vi "Load Slave Configuration.vi"(8 "error in":errorcluster) -> (0 "error out":errorcluster, 1 "JointMapping":T1, 2 "hw interface":T4, 3 "kinematic parameters":T3)   [LabVIEW 2013]
uses:
  <vilib>/robotics/Kinematics/Link/Joint Type.ctl
  Telemanipulation/Grips Robot/JointMapping.ctl
  <vilib>/NI/GXML/_subVIs/GXML SearchParser/Search Parser.vi
  <vilib>/NI/GXML/GXML.lvlib
  <vilib>/robotics/Kinematics/Link/NI_Robotics_Link.lvclass
  Telemanipulation/Grips Robot/Grips Robot.lvclass
panel:
  out "file path":path
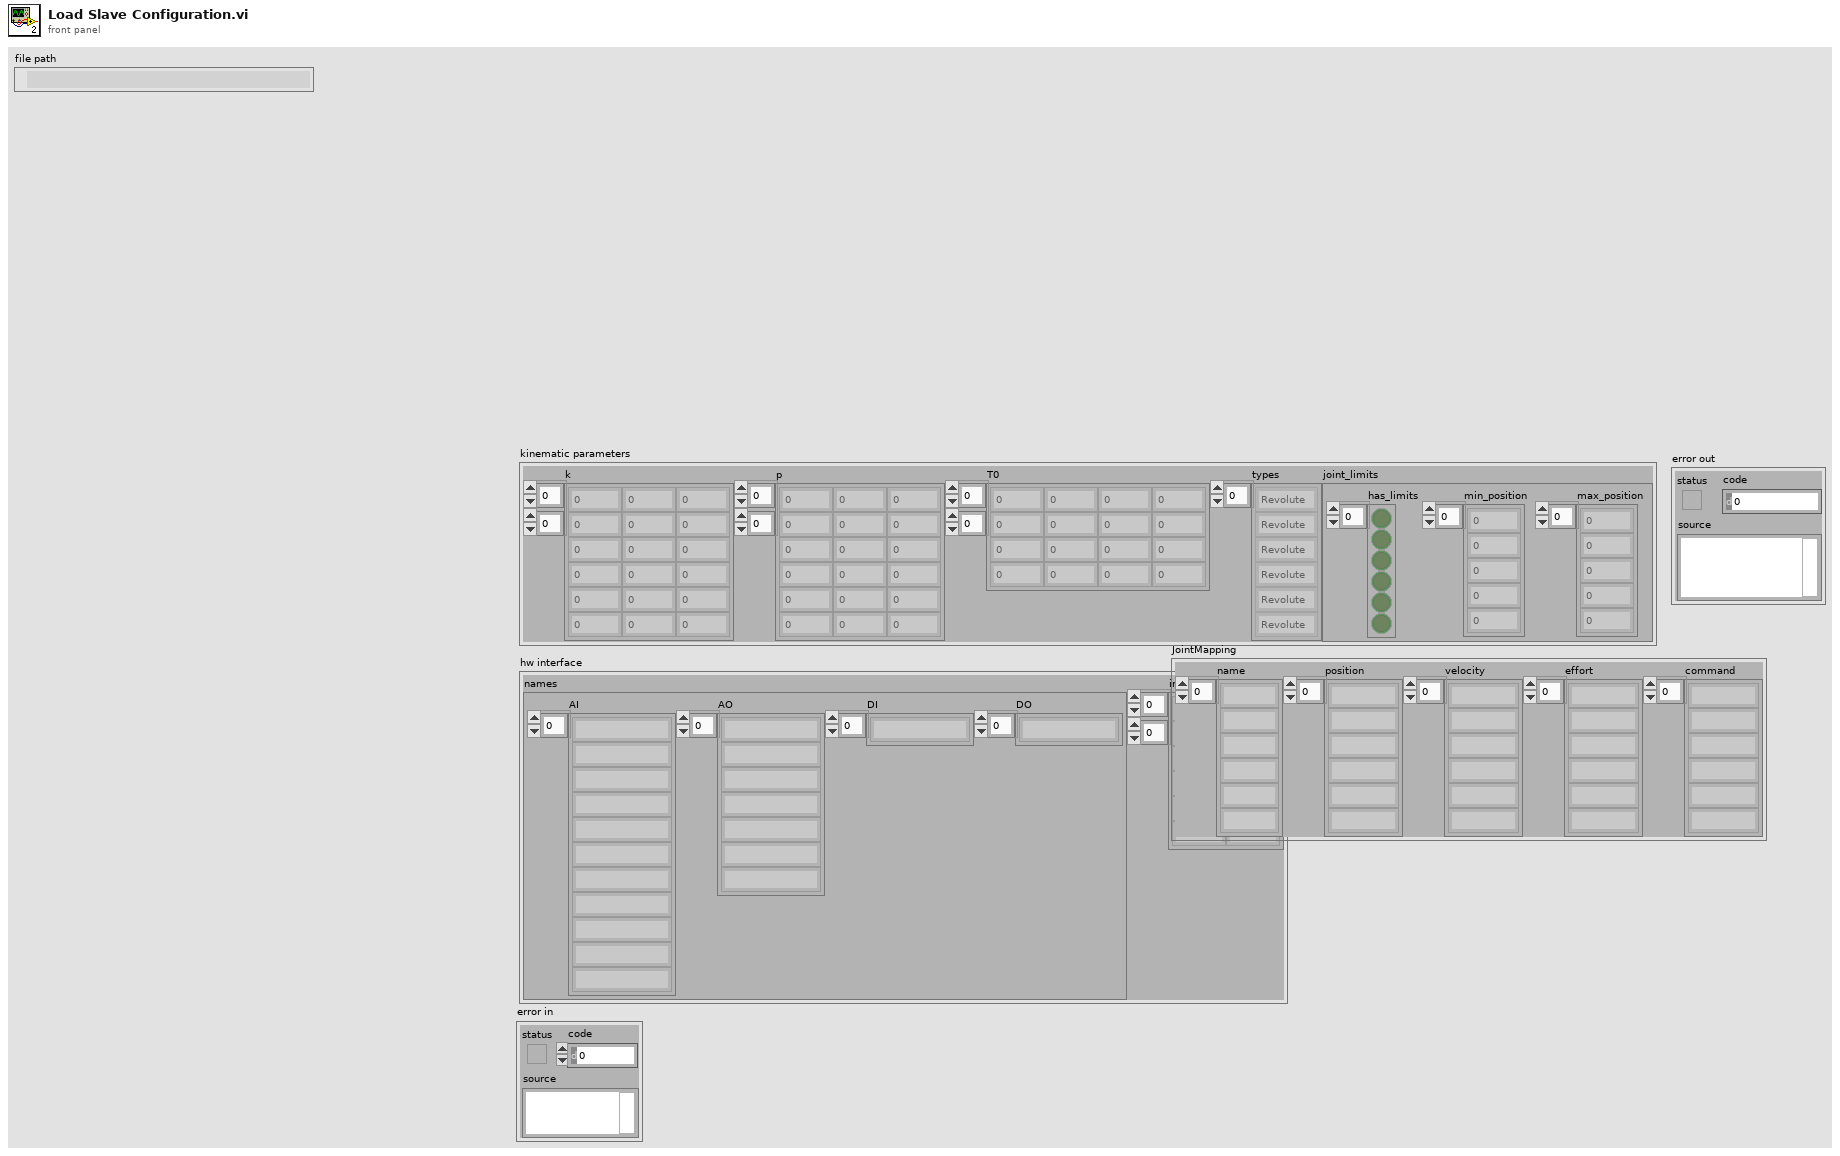
[diagram p1: front panel]
types:
  T1 = typedef "Grips Robot.lvclass/JointMapping.ctl" = cluster{"name":string[], "position":string[], "velocity":string[], "effort":string[], "command":string[]}
  T2 = typedef "NI_Robotics_Link.lvclass/Joint Type.ctl" = enum16{"Revolute", "Prismatic"}
  T3 = cluster{"k":sgl[][], "p":sgl[][], "T0":sgl[][], "types":T2[], "joint_limits":cluster{"has_limits":bool[], "min_position":sgl[], "max_position":sgl[]}}
  T4 = cluster{"names":cluster{"AI":string[], "AO":string[], "DI":string[], "DO":string[]}, "interpolation_coeff":sgl[][]}
  T5 = cluster{"name":string[], "position":string[], "velocity":string[], "effort":string[], "command":string[]}
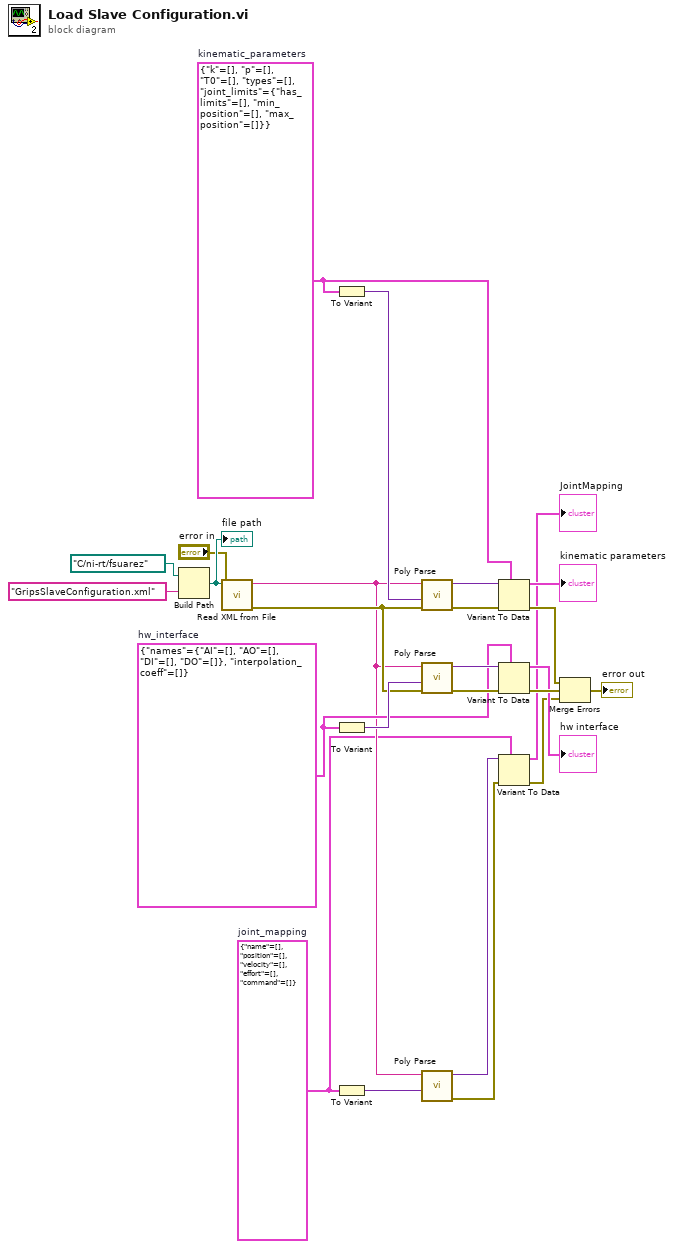
[diagram p0: block diagram]
diagram:
  w3 = T5 {"name"=[], "position"=[], "velocity"=[], "effort"=[], "command"=[]}  # joint_mapping
  w11 = T4 {"names"={"AI"=[], "AO"=[], "DI"=[], "DO"=[]}, "interpolation_coeff"=[]}  # hw_interface
  w12 = T3 {"k"=[], "p"=[], "T0"=[], "types"=[], "joint_limits"={"has_limits"=[], "min_position"=[], "max_position"=[]}}  # kinematic_parameters
  n1 = Build Path(base path=path "C:/ni-rt/fsuarez", name or relative path="GripsSlaveConfiguration.xml") -> (appended path=w23:path)
  "file path" <- w23
  n2 = call <vilib>:"Read XML from File.vi"("error in"="error in", "XML File Path"=w23) -> ("error out"=w13:errorcluster, "XML String Out"=w5:string)  [unwired: 8 in]
  n3 = To Variant(anything=w12) -> (Variant=w22:variant)
  n4 = To Variant(anything=w11) -> (Variant=w20:variant)
  n5 = To Variant(anything=w3) -> (Variant=w6:variant)
  n6 = call-poly <vilib>:"Poly Parse.vi"("error in"=w13, "TypeDesc"=w22, "XML String In"=w5) -> ("error out"=w19:errorcluster, "Parsed Data"=w21:variant)  [unwired: 7 in]
  n7 = call-poly <vilib>:"Poly Parse.vi"("error in"=w13, "TypeDesc"=w20, "XML String In"=w5) -> ("error out"=w16:errorcluster, "Parsed Data"=w17:variant)  [unwired: 7 in]
  n8 = call-poly <vilib>:"Poly Parse.vi"("TypeDesc"=w6, "XML String In"=w5) -> ("error out"=w7:errorcluster, "Parsed Data"=w8:variant)  [unwired: 8 in]
  n9 = Variant To Data(error in=w19, type=w12, Variant=w21) -> (data=→"kinematic parameters":T3, error out=w18:errorcluster)
  n10 = Variant To Data(error in=w16, type=w11, Variant=w17) -> (data=→"hw interface":T4, error out=w15:errorcluster)
  n11 = Variant To Data(error in=w7, type=w3, Variant=w8) -> (data=→"JointMapping":T5, error out=w4:errorcluster)
  n12 = Merge Errors(w18, w15, w4) -> (→"error out":errorcluster)
